vi "Flush Check.vi"(8 "error in (no error)":errorcluster, 11 "TDMS in":refnum<class "TDMS.lvclass">) -> (0 "error out":errorcluster, 3 "TDMS out":refnum<class "TDMS.lvclass">)   [LabVIEW 2019, in "TDMS.lvlib" / "TDMS.lvclass"]
uses:
  TDMS.lvclass
  TDMS.lvclass/TDMS.ctl
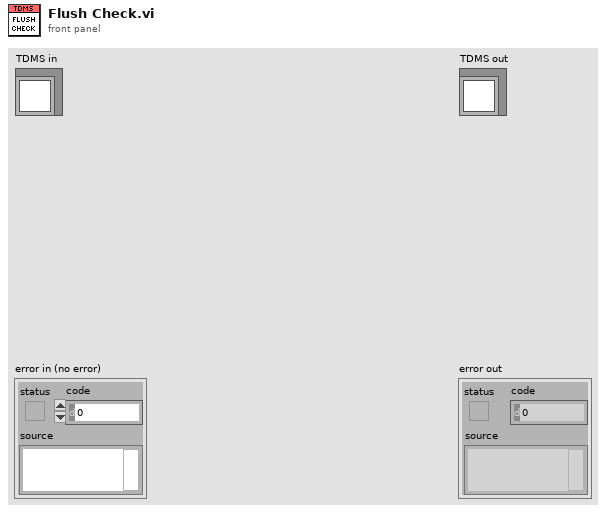
[diagram p1: front panel]
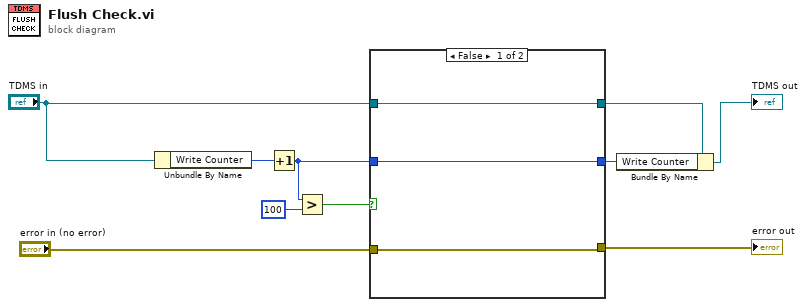
[diagram p0: block diagram]
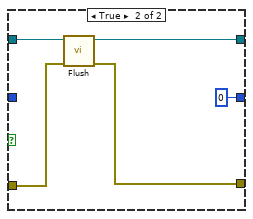
[diagram p2: hidden frame]
diagram:
  n1 = Unbundle By Name("TDMS in") -> ("Write Counter"=w10:i32)
  n2 = Increment(x=w10) -> (x+1=w6:i32)
  n3 = Greater?(x=w6, y=100) -> (0:w8:bool)
  n4 = case shown="False" w8 {
    tunnel: "TDMS in" -> [w12 w17]
    tunnel: w6 -> [w13 _]
    tunnel: [w13 0] -> w5
    tunnel: [w12 w16] -> w4
    tunnel: "error in (no error)" -> [w11 w15]
    tunnel: [w11 w14] -> w1
    frame False {
    }
    frame True {
      n5 = call-dynamic "Flush.vi"("error in"=w15, "TDMS in"=w17) -> ("error out"=w14:errorcluster, "TDMS out"=w16:refnum<class "TDMS.lvclass">)  [unwired: 8 in]
    }
  }
  "error out" <- w1
  n6 = Bundle By Name(cluster=w4, "Write Counter"=w5) -> (→"TDMS out":refnum<class "TDMS.lvclass">)
